vi "loadICOS.vi"() -> ()   [LabVIEW 2012]
panel:
  out "appended path":path
  out "path out":path
  out "String":string
  in  "Array":string[](array[string])=["\\hexa\\FLST08", "\\hexa\\FLST09", "\\hexa\\FLST10", "\\hexa\\FLST11", "\\hexa\\FLST12", "\\hexa\\FLST13", "\\hexa\\FLST14", "\\hexa\\FLST15", "\\hexa\\FLST21", "\\hexa\\FLST22", "\\hexa\\FLST27", "\\hexa\\FLST28"]
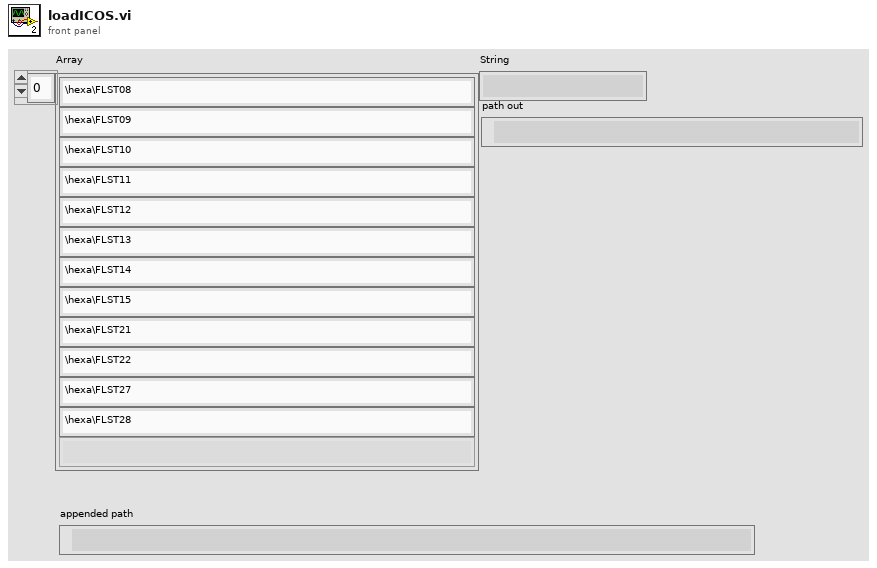
[diagram p1: front panel]
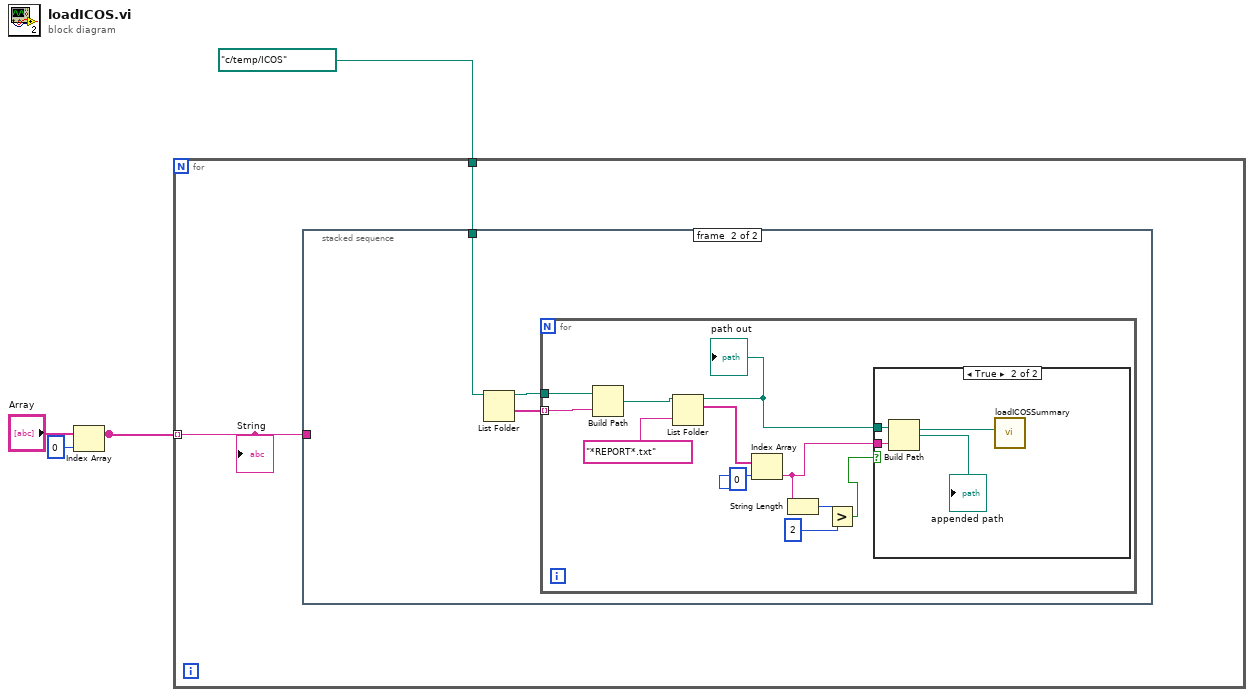
[diagram p0: block diagram]
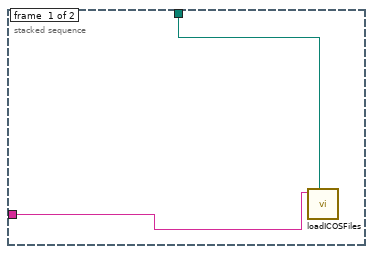
[diagram p2: hidden frame]
diagram:
  n1 = Index Array(array="Array", index=0) -> ()  [unwired: 1 out]
  n2 = for {
    tunnel: path "c:/temp/ICOS" ("path") -> [w5]
    tunnel: "Array" -> [w4] mode=indexing
    n3 = stacked-sequence {
      tunnel: w5 -> [w6 w10]
      tunnel: w4 -> [w7 _]
      frame #0 {
        n4 = call "loadICOSFiles.vi"("working directory"=w6, "Path"=w7) -> ()  [unwired: 10 in]
      }
      frame #1 {
        n5 = List Folder(path=w10) -> (path out=w9:path, folder names=w8:string[])  [unwired: 3 in, 2 out]
        n6 = for {
          tunnel: w9 -> [w21]
          tunnel: w8 -> [w20] mode=indexing
          n7 = Build Path(base path=w21, name or relative path=w20) -> (appended path=w18:path)
          n8 = List Folder(path=w18, pattern="*REPORT*.txt") -> (path out=w15:path, filenames=w17:string[])  [unwired: 2 in, 2 out]
          "path out" <- w15
          n9 = Index Array(array=w17, index=0) -> (element=w14:string)
          n10 = String Length(string=w14) -> (length=w13:i32)
          n11 = Greater?(x=w13, y=2) -> (0:w11:bool)
          n12 = case shown="True" w11 {
            tunnel: w15 -> [_ w24]
            tunnel: w14 -> [_ w22]
            frame False {
            }
            frame True {
              n13 = Build Path(base path=w24, name or relative path=w22) -> (appended path=w23:path)
              "appended path" <- w23
              n14 = call "loadICOSSummary.vi"("file path (dialog if empty)"=w23) -> ()  [unwired: 10 in, 1 out]
            }
          }
        }
      }
    }
    "String" <- w4
  }
